vi "XML Build Poll Request(1).vi"(2 "XML-Message alt":string, 3 "EVID-Nummer":i32=1) -> (0 "Attribut Name":string, 7 "XML-Message neu":string)   [LabVIEW 2020, in "FT-IR.lvlib" / "TOOLweb Interface.lvlib" / "TOOLweb Interface Hilfs-VIs.lvlib"]
doc: "Fügt an die bisher aufgebauten XML-Poll-Request-Zeilen \"XML-Message alt\" eine Poll-Request-Zeile hinzu, die eine Variable \"EVID-Nummer\" anfordert.\n\nDer Ausgang \"Attribut Name\" wird zu einem auf gleicher Höhe liegendem XML-Parser verbunden, der damit keine weiteren Informationen benötigt.\n\nDer Ausgangs-String \"XML-Message neu\" wird an ein weiteres XML-Build-VI oder an das abschließende \"XML Build Poll Request Frame\" übergeben, das allen Zeilen gemeinsam mit dem Start-Tag <PollRequest> und dem End-Tag </PollRequest> den Rahmen für eine einzige und damit schnelle XML-Anfrage gibt."
uses:
  TOOLweb Interface Hilfs-VIs.lvlib
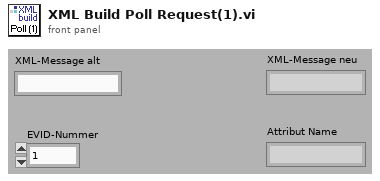
[diagram p1: front panel]
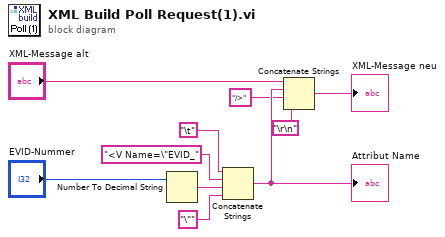
[diagram p0: block diagram]
diagram:
  n1 = Number To Decimal String(number="EVID-Nummer") -> (decimal integer string=w8:string)  [unwired: 1 out]
  n2 = Concatenate Strings("\t", "<V Name=\"EVID_" ("Daten (Eingang)"), w8, "\"" ("Daten (Eingang)")) -> (w4:string)
  "Attribut Name" <- w4
  n3 = Concatenate Strings("XML-Message alt", w4, "/>" ("Daten (Eingang)"), "\r\n") -> (→"XML-Message neu":string)
